vi "linescan.vi"(5 "DAQ analog output":tag="Dev1/ao0", 6 "duration":dbl=0.1 format="%#_6p", 7 "DAQ sampling rate":dbl=100000000.0 format="%#_6p", 8 "error in (no error)":errorcluster, 9 "#counter bins":i32=100, 10 "analog output voltage2":dbl format="%.3f", 11 "analog output voltage1":dbl format="%.3f") -> (0 "error out":errorcluster, 3 "histogram plot":dbl[](graph)=[0.0, 0.0, 3000.0, 4000.0, 0.0, 0.0, 1000.0, 0.0, 0.0, 3000.0, 0.0, 1000.0, 0.0, 2000.0, 0.0, 0.0, 1000.0, 0.0, 2000.0, 1000.0, 4000.0, 0.0, 0.0, 0.0, 0.0, 0.0, 8000.0, 0.0, 0.0, 0.0, 1000.0, 0.0, 5000.0, 0.0, 0.0, 0.0, 0.0, 2000.0, 5000.0, 0.0, 0.0, 0.0, 0.0, 3000.0, 3000.0, 0.0, 0.0, 0.0, 1000.0, 2000.0, 1000.0, 0.0, 0.0, 1000.0, 0.0, 1000.0, 2000.0, 0.0, 2000.0, 0.0, 0.0, 0.0, 2000.0, 0.0, 0.0, 0.0, 0.0, 3000.0, 1000.0, 0.0, 0.0, 0.0, 1000.0, 3000.0, 3000.0, 0.0, 0.0, 2000.0, 0.0, 6000.0, 0.0, 1000.0, 1000.0, 0.0, 2000.0, 4000.0, 0.0, 0.0, 0.0, 0.0, 0.0, 0.0, 0.0, 1000.0, 0.0, 0.0, 2000.0, 2000.0, 0.0, 0.0])   [LabVIEW 2014]
uses:
  global_channels.vi
panel:
  in  "filter":bool=TRUE
  # "[s]"
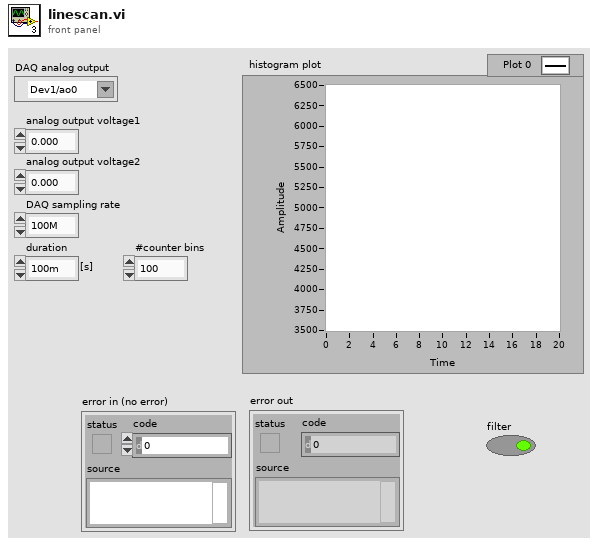
[diagram p1: front panel]
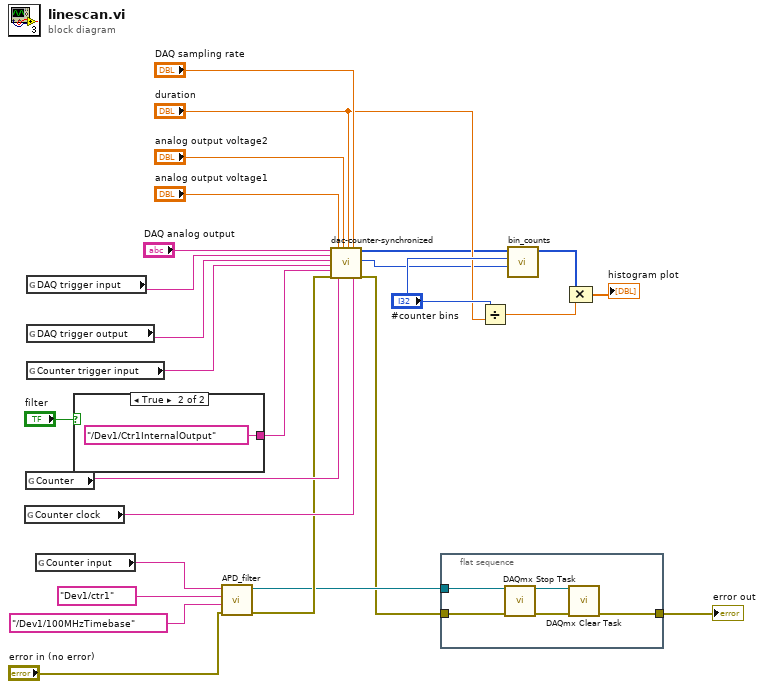
[diagram p0: block diagram]
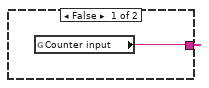
[diagram p2: hidden frame]
diagram:
  n1 = global read "global_channels.vi" "Counter clock"() -> (w11:tag)
  n2 = global read "global_channels.vi" "Counter"() -> (w12:tag)
  n3 = global read "global_channels.vi" "DAQ trigger input"() -> (w15:tag)
  n4 = global read "global_channels.vi" "DAQ trigger output"() -> (w14:tag)
  n5 = global read "global_channels.vi" "Counter trigger input"() -> (w13:tag)
  n6 = global read "global_channels.vi" "Counter input"() -> (w10:tag)
  n7 = case shown="True" "filter" {
    tunnel: [w27 tag "/Dev1/Ctr1InternalOutput" ("source of ticks")] -> w2
    frame False {
      n8 = global read "global_channels.vi" "Counter input"() -> (w27:tag)
    }
    frame True {
    }
  }
  n9 = call "APD_filter.vi"("error in"="error in (no error)", "source of ticks"=tag "/Dev1/100MHzTimebase", "counter_filter"=tag "Dev1/ctr1", "APD signal"=w10) -> ("error out"=w7:errorcluster, "filtered APD"=w6:refnum<k21>)  [unwired: 2 in]
  n10 = call "dac-counter-synchronized.vi"("DAQ analog output"="DAQ analog output", "DAQ trigger input"=w15, "DAQ trigger output"=w14, "Counter trigger input"=w13, "counter input"=w2, "error in (no error)"=w7, "analog output voltage1"="analog output voltage1", "counter"=w12, "analog output voltage2"="analog output voltage2", "Duration"="duration", "DAQ sampling rate"="DAQ sampling rate", "Clock source"=w11) -> ("time tags"=w17:u32[], "clock cycles"=w16:i32, "error out"=w5:errorcluster)  [unwired: 4 in, 1 out]
  n11 = flat-sequence {
    tunnel: w6 -> [w31]
    tunnel: w5 -> [w30]
    tunnel: [w29] -> w4
    frame #0 {
      n12 = call <vilib>:"DAQmx Stop Task.vi"("task/channels in"=w31, "error in"=w30) -> ("task out"=w33:refnum<k21>, "error out"=w32:errorcluster)  [unwired: 12 in]
      n13 = call <vilib>:"DAQmx Clear Task.vi"("task in"=w33, "error in"=w32) -> ("error out"=w29:errorcluster)  [unwired: 13 in]
    }
  }
  n14 = Divide(x="#counter bins", y="duration") -> (x/y=w24:dbl)
  n15 = call "bin_counts.vi"("#clock cycles"=w16, "#bins"="#counter bins", "counter timetag list"=w17) -> ("histogram"=w23:i32[])  [unwired: 4 in, 3 out]
  n16 = Compound Arithmetic op=MULTIPLY(w23, w24) -> (→"histogram plot":dbl[])
  "error out" <- w4
